vi "fusion_receiver.vi"() -> ()   [LabVIEW 2015]
panel:
  out "Received Data":dbl(graph)
  in  "Stop":bool
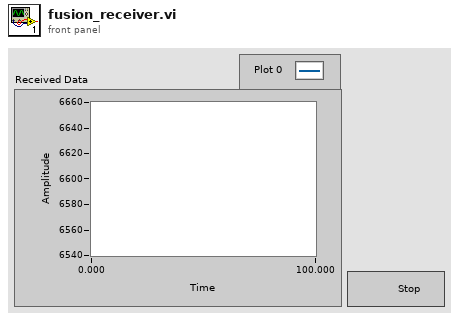
[diagram p1: front panel]
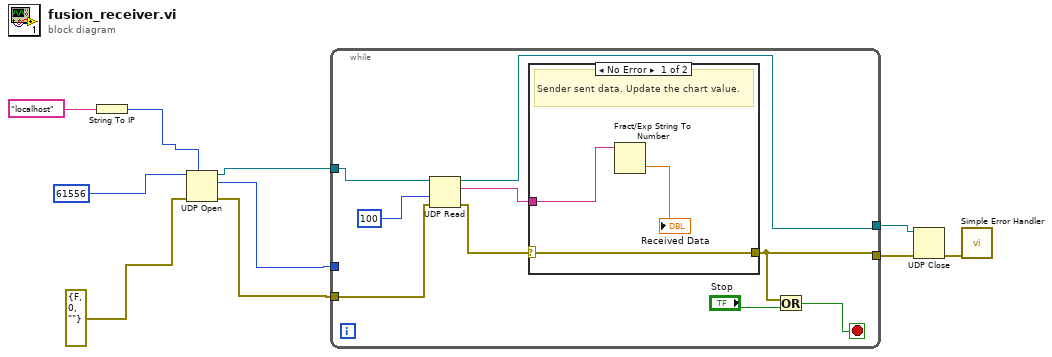
[diagram p0: block diagram]
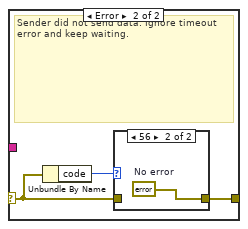
[diagram p2: hidden frame]
diagram:
  n1 = String To IP(1:"localhost" ("name")) -> (0:w9:u32)
  n2 = UDP Open(7:w9, 8:errorcluster {"status"=FALSE, "code"=0, "source"=""} ("error in (no error)"), 11:u16 61556 ("port")) -> (port=w8:refnum<k16>, 0:w5:errorcluster, 2:w7:u16)  [unwired: 2 in]
  n3 = while {
    tunnel: w8 -> [w19]
    tunnel: w7 -> [_]
    tunnel: w5 -> [w17]
    tunnel: [w15] -> w3
    tunnel: [w14] -> w2
    stop <- w13 stop-if-true
    n4 = UDP Read(connection ID=w19, timeout ms (25000)=100, 8:w17) -> (data out=w12:string, error out=w11:errorcluster, 3:w15:refnum<k16>)  [unwired: 1 in, 2 out]
    n5 = case shown="No Error" w11 {
      selector: w11 -> [w22 w24]
      tunnel: w12 -> [w21 _]
      tunnel: [w22 w23] -> w14
      frame No Error {
        # "Sender sent data. Update the chart value."
        n6 = Fract/Exp String To Number(string=w21) -> (number=→"Received Data":dbl)  [unwired: 3 in, 1 out]
      }
      frame Error {
        # "Sender did not send data. Ignore timeout error and keep waiting."
        n7 = Unbundle By Name(w24) -> ("code"=w25:i32)
        n8 = case shown="56" w25 {
          tunnel: w24 -> [w26 _]
          tunnel: [w26 w27] -> w23
          frame Default {
          }
          frame 56 {
            w27 = errorcluster {"status"=FALSE, "code"=0, "source"=""}  # No error
          }
        }
      }
    }
    n9 = Or(x=w14, y="Stop") -> (x .or. y?=w13:bool)
  }
  n10 = UDP Close(connection ID=w3, 8:w2) -> (error out=w4:errorcluster)  [unwired: 1 out]
  n11 = call <vilib>:"Simple Error Handler.vi"("error in (no error)"=w4) -> ()  [unwired: 1 in, 8 out]
